vi "401_Audit_Report.vi"() -> (0 "error Out":errorcluster)   [LabVIEW 2015]
uses:
  Utilities/TypeDefs/401_Audit_Activity.ctl
  Utilities/TypeDefs/401_Audit_States.ctl
  <vilib>/addons/database/Connection.llb/Conn ObjectReference.ctl
  System Settings/Modules/LV2GActions.ctl
  <vilib>/Utility/miscctls.llb/LVPointTypeDef.ctl
  <vilib>/Utility/miscctls.llb/LVRowAndColumnUnsignedTypeDef.ctl
  <vilib>/addons/database/NI_Database_API.lvlib
panel:
  in  "Decending":bool caption="Asc/Des"
  in  "Tab Processing":enum32{"Page 1"}(tab)
  in  "VS":bool=TRUE
  in  "Export":bool
  in  "Tab Control":enum32{"Date", "User Name"}(tab)
  in  "Start Date":timestamp format="%<%H:%M:%S\n%Y/%m/%d>T"
  in  "End Date":timestamp format="%<%H:%M:%S\n%Y/%m/%d>T"
  in  "User":u16(ring) items=["Admin", "Supervisor", "Operator"]
  in  "Save":bool
  in  "Multicolumn Listbox":i32(listbox)
  in  "Activity":T1=enum."User show functionality for Info"
  in  "Previous Value":dbl
  in  "Current Value":dbl
  out "Date,Time":string
  in  "USER ID":string="Rahul"
  in  "Back":bool
  in  "Boolean":bool
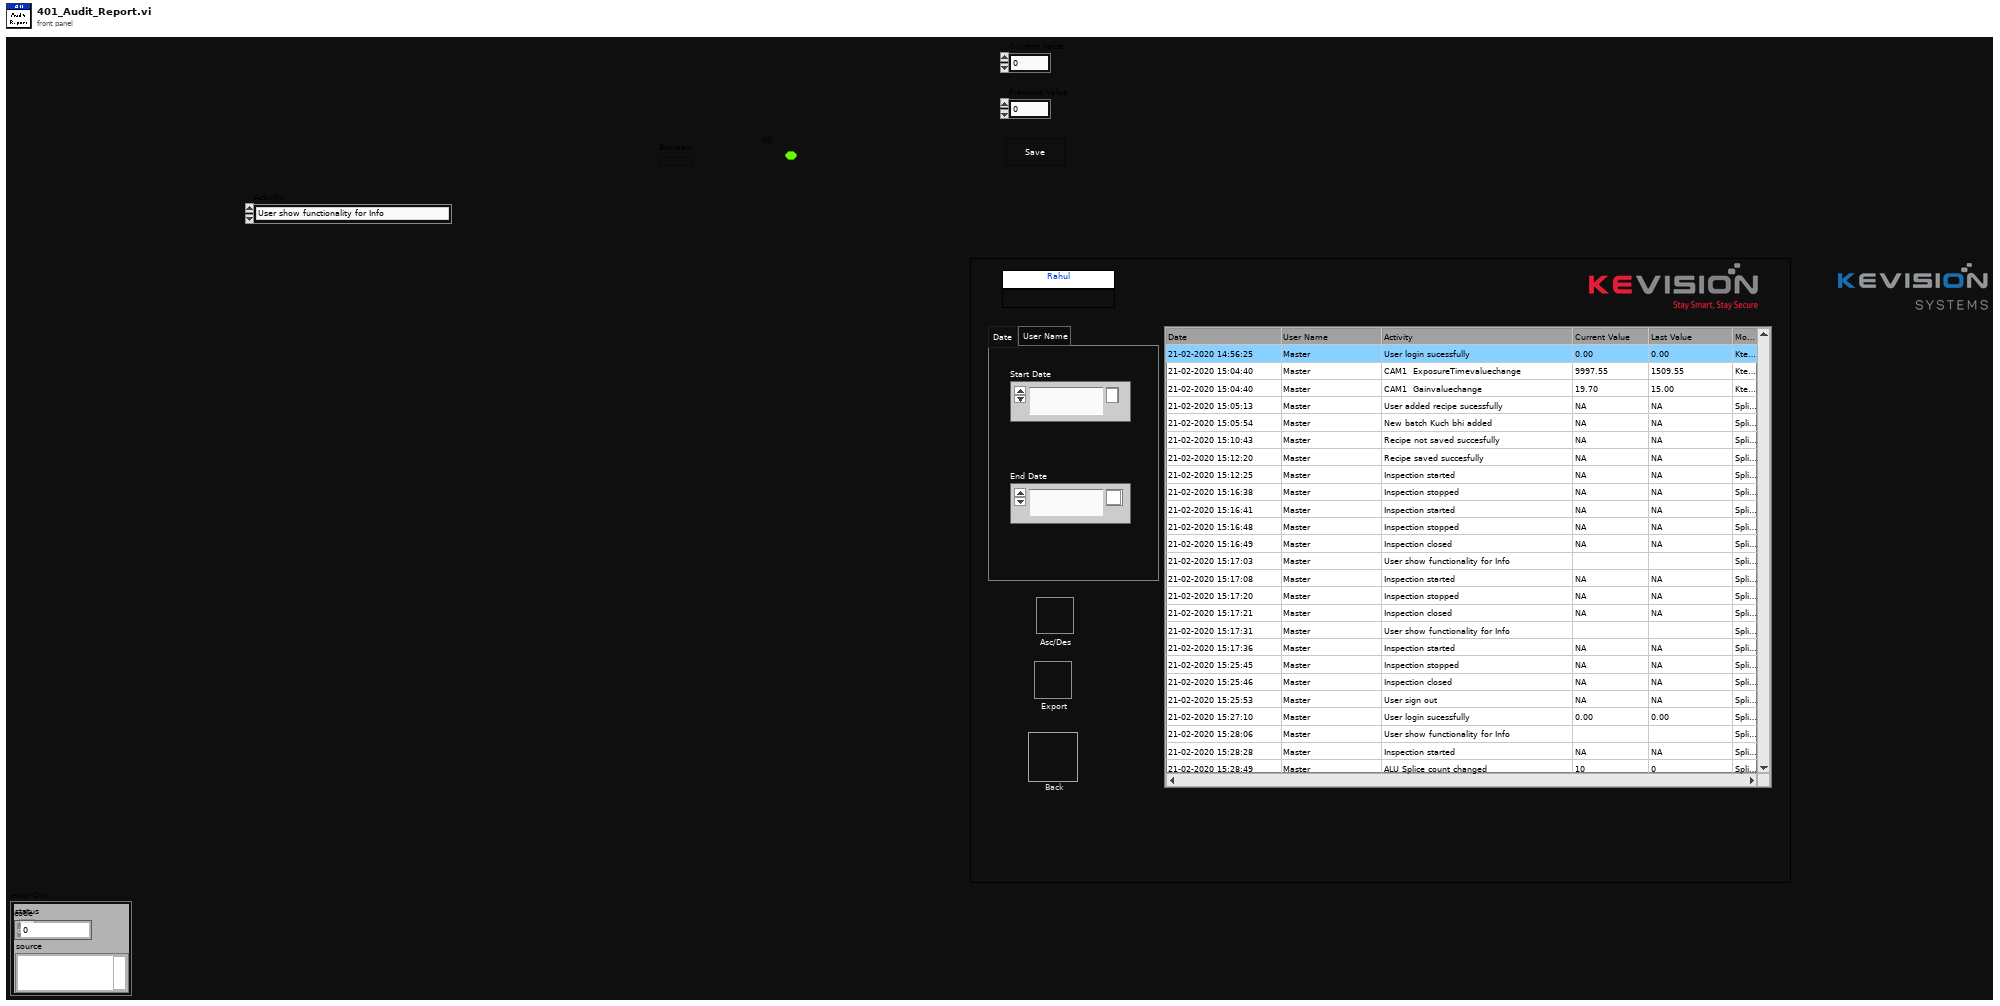
[diagram p1: front panel]
types:
  T1 = typedef "401_Audit_Activity.ctl" = enum16{"User login sucessfully", "User login fail", "User lock", "User sign out", "User added succesfully", "User edit succesFully", "User delete succesfully", "Reset password", "Forgot Password", "User change security policy", "User change user rights", "User allowed functionality for inspection", "User allowed  functionality for recipe", "User allowed functionality for teach", "User allowed  for user management", "User allowed for camera settings", "User allowed functionality for Hardware Check", "User allowed functionality for printer settings", "User allowed functionality for server settings", "User allowed  for third party settings", "User allowed  for System settings", "User allowed functionality For Test I/O", "User allowed and show functionality For Fault Images", "User allowed functionality for Production Report", "User allowed functionality for Audit Report", "User allowed functionality for Help", "User allowed functionality for  Info", "User show functionality for Inspection", "User show functionality for Teach", "User show functionality for Recipe", "User show functionality for User Management", "User show functionality for Camera Settings", "User show functionality for Hardware Check", "User show functionality for printer Settings", "User show functionality  for Server Settings", "User show functionality for Third party Settings", "User show functionality for System settings", "User show functionality for Test I/O", "User show functionality for Fault Images", "User show functionality for Production Report", "User show functionality for Audit Report", "User show functionality for Help", "User show functionality for Info", "User update Security Policy", "User added Recipe sucessfully", "User delete Recipe sucessfully", "User rename Recipe sucessfully", "User save Camera Settings sucessfully ", "User Close with out save", "User change Brightness", "User change Exposure Time", "User change Gain Value", "User change Saturation", "User change Gamma", "User change Sharpness", "User change Hue", "User change White Balance", "User change  Comport ", "User save Test I/o settings sucessfully", "User close with out saving ", "User change Light Timing ", "User change Light Flash ", "Camera Ready", "User change Inactive Period ", "User change Grab Delay", "User change Timed Output", "User change No Of Track", "User change Output Polarity ", "User chnage Output Timing", "User change Track Output ", "User Taught sucessfully", "User close with out  Taught.", "User could not able To Add User", "User could not Delete", "User could not Updated", "User could not change Security Policy", "User could not change User Rights"}
  T2 = typedef "401_Audit_States.ctl" = enum16{"Intialize", "UpdateControls", "Save", "User Interface", "Finalize", "View User Data", "View Date time Data", "Add Audit Data", "Decending", "Ascending", "Export To Html", "UpdateFPCControls", "Quit"}
  T3 = typedef "NI_Database_API.lvlib/Conn ObjectReference.ctl" = refnum<k1>
  T4 = cluster{"states":T2, "error in":cluster{"status":bool, "Error in":i32, "source":string}, "Save Data":cluster{"Current Value":dbl, "Previous Value":dbl, "Activity Name":string, "Camera Name":string}, "DB_Ref_In":T3, "Multicolumn Listbox":refnum<vi>, "Read Data":string[][], "Selecteduser":string}
  T5 = typedef "LV2GActions.ctl" = enum16{"Read", "Write", "Current", "Update", "UpdateSystemSettings", "UpdateModel"}
  T6 = typedef "LVPointTypeDef.ctl" = cluster{"Horizontal":i16, "Vertical":i16}
  T7 = cluster{"UserName":string, "Group Level":u16, "Theme":u16, "Software Type":u16, "System Language":u16, "Master":bool, "Recipe":string, "Batch":string, "Simulate":bool, "Trigger Activation":u16, "DateFormat":u16, "HardwareTest":bool}
  T8 = enum8{"Enabled", "Disabled", "Disabled and Grayed Out"}
  T9 = typedef "LVRowAndColumnUnsignedTypeDef.ctl" = cluster{"Row":u32, "Column":u32}
  T10 = enum16{"Read", "Current", "UpdateRecipiePath", "UpdateBatchPath"}
  T11 = cluster{"status":bool, "Error in":i32, "source":string}
  T12 = cluster{"BasePath":path, "RecipiePath":path, "BatchPath":path}
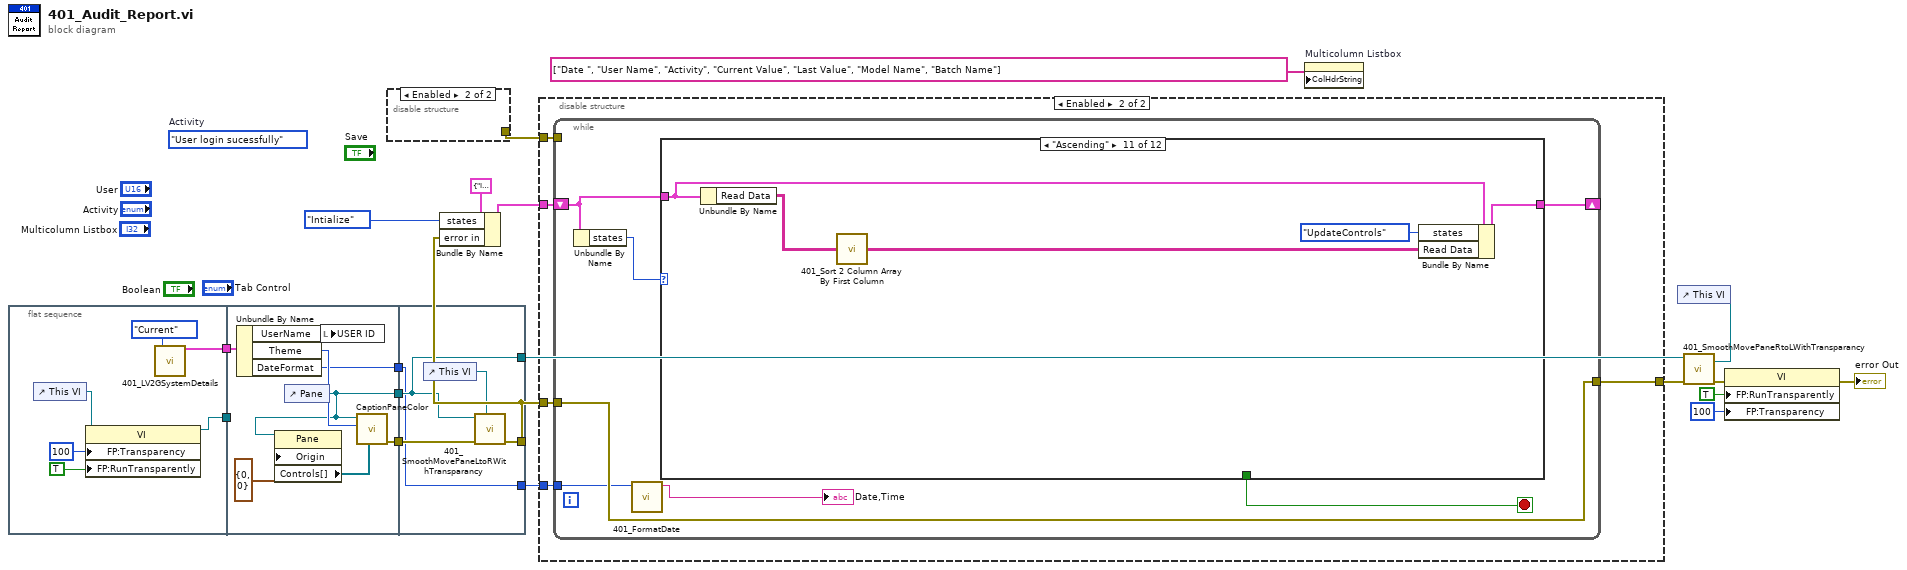
[diagram p0: block diagram]
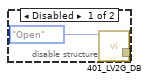
[diagram p2: hidden frame]
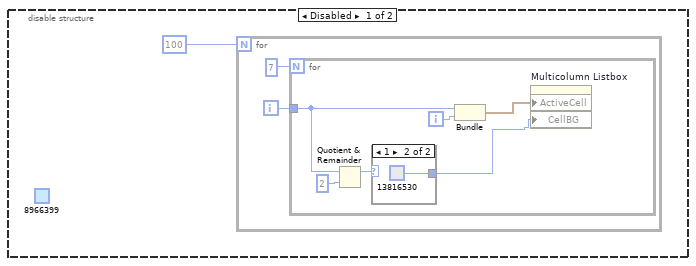
[diagram p3: hidden frame]
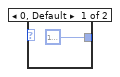
[diagram p4: hidden frame]
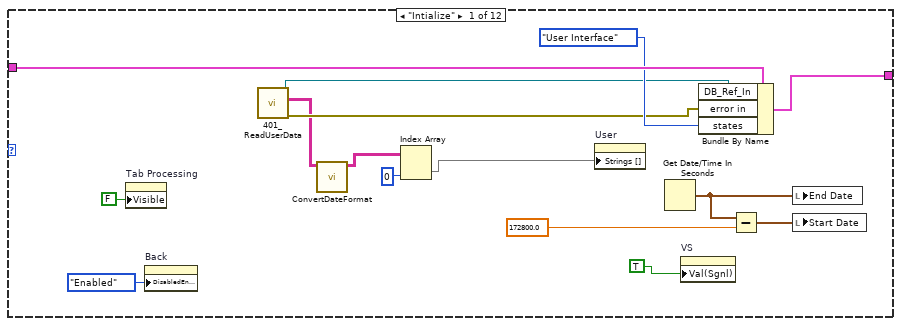
[diagram p5: hidden frame]
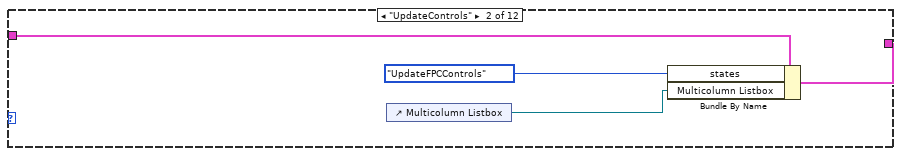
[diagram p6: hidden frame]
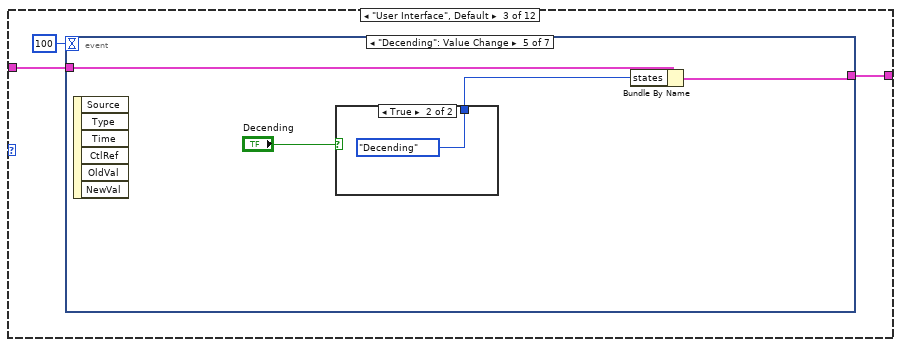
[diagram p7: hidden frame]
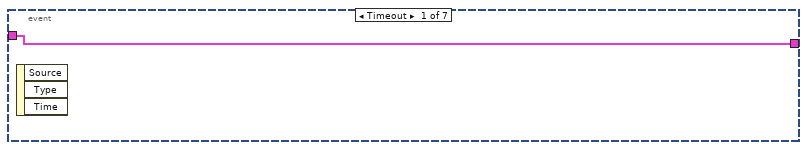
[diagram p8: hidden frame]
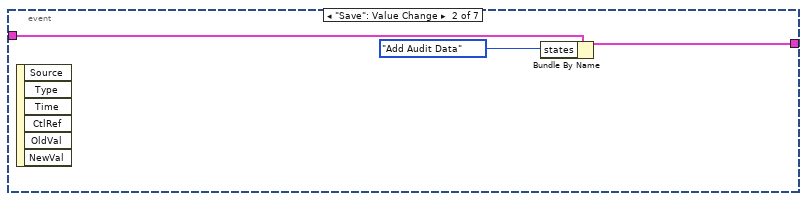
[diagram p9: hidden frame]
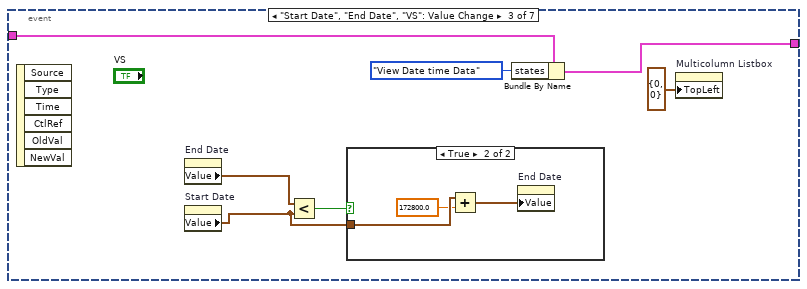
[diagram p10: hidden frame]
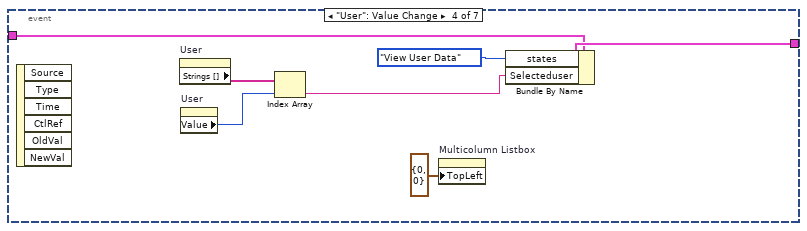
[diagram p12: hidden frame]
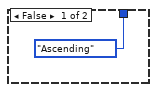
[diagram p13: hidden frame]
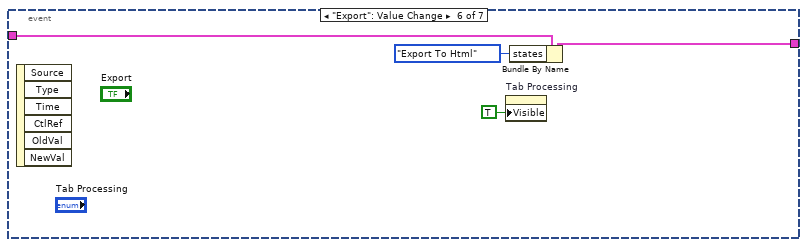
[diagram p14: hidden frame]
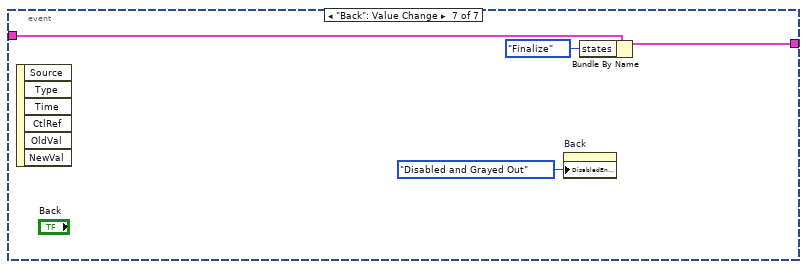
[diagram p15: hidden frame]
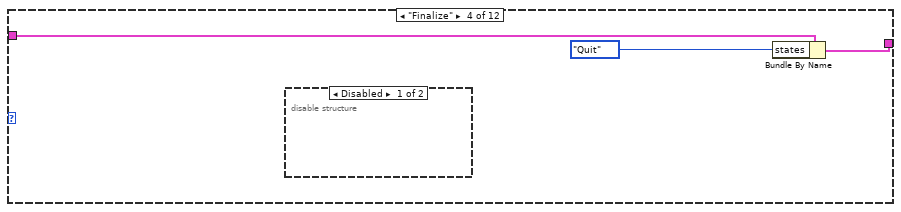
[diagram p16: hidden frame]
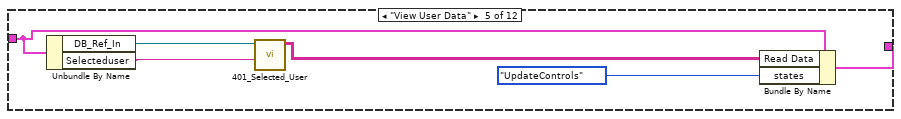
[diagram p18: hidden frame]
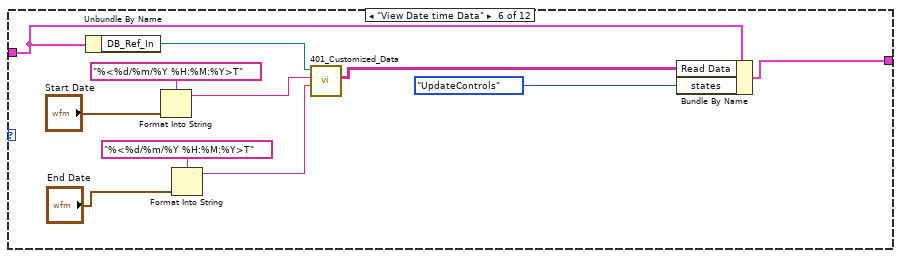
[diagram p19: hidden frame]
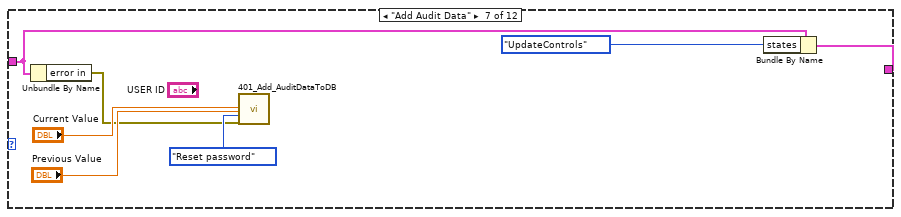
[diagram p20: hidden frame]
diagram:
  (unwired) 401_Audit_Activity."User login sucessfully"  # Activity
  n1 = flat-sequence {
    tunnel: [w22] -> w13
    tunnel: [w20] -> w11
    tunnel: w13 -> [_]
    tunnel: [w33] -> w12
    tunnel: w11 -> [w30]
    tunnel: [w27] -> w5
    tunnel: [w26] -> w2
    tunnel: [w37] -> w8
    tunnel: w12 -> [w36]
    tunnel: w5 -> [w35]
    tunnel: [w35] -> w4
    tunnel: [w34] -> w3
    tunnel: w2 -> [w34]
    frame #0 {
      n2 = control-ref of="This VI"() -> (w25:refnum<vi>)
      n3 = property class="VI"(reference=w25, "FP:Transparency"=u8 100 ("Front Panel Window:Transparency"), "FP:RunTransparently"=TRUE ("Front Panel Window:Run VI Transparently")) -> (reference out=w22:refnum<vi>)  [unwired: 1 in, 1 out]
      n4 = call "401_LV2GSystemDetails.vi"("R/W/C"=LV2GActions."Current") -> ("DataOut"=w20:T7)  [unwired: 17 in, 1 out]
    }
    frame #1 {
      n5 = Unbundle By Name(w30) -> ("UserName"=w28:string, "Theme"=w29:u16, "DateFormat"=w26:u16)
      n6 = control-ref of="Pane"() -> (w27:refnum<vi>)
      n7 = property class="Pane"(reference=w27, "Origin"=T6 {"Horizontal"=0, "Vertical"=0}) -> ("Controls[]"=w32:refnum<vi>[])  [unwired: 1 in, 2 out]
      n8 = local write "USER ID"(w28) -> ()
      n9 = call "CaptionPaneColor.vi"("Controls[]"=w32, "NewVal"=w29, "Pane in"=w27) -> ("error out"=w33:errorcluster)  [unwired: 8 in]
    }
    frame #2 {
      n10 = control-ref of="This VI"() -> (w38:refnum<vi>)
      n11 = call "401_SmoothMovePaneLtoRWithTransparancy.vi"("VI in"=w38, "error in (no error)"=w36, "Pane in"=w35) -> ("error out"=w37:errorcluster)  [unwired: 7 in, 1 out]
    }
  }
  n12 = disable-structure shown="Enabled" {
    disable-tunnel: [w39 _] -> w1
    frame Disabled {
      n13 = call "401_LV2G_DB.vi"("Action"=enum16{"Open", "Read", "Close"}."Open") -> ("error out"=w39:errorcluster)  [unwired: 9 in, 1 out]
    }
    frame Enabled {
    }
  }
  n14 = Bundle By Name(cluster=T4 {"states"=enum."Intialize", "error in"={"status"=FALSE, "Error in"=0, "source"=""}, "Save Data"={"Current Value"=0.0, "Previous Value"=0.0, "Activity Name"="", "Camera Name"=""}, "DB_Ref_In"=refnum, "Multicolumn Listbox"=refnum, "Read Data"=[], "Selecteduser"=""} ("input cluster"), "states"=401_Audit_States."Intialize", "error in"=w8) -> (w14:T4)
  n15 = disable-structure shown="Enabled" {
    disable-tunnel: w14 -> [_ w56]
    disable-tunnel: w8 -> [_ w55]
    disable-tunnel: [_ w54] -> w17
    disable-tunnel: w3 -> [_ w53]
    disable-tunnel: w1 -> [_ w52]
    frame Disabled {
      (unwired) u32 8966399
      n16 = for {
        N: 100 -> [_]
        i -> [w42]
        n17 = for {
          N: 7 -> [_]
          tunnel: w42 -> [w48]
          i -> [w49]
          n18 = Quotient & Remainder(x=w48, y=2) -> (x-y*floor(x/y)=w46:i32)  [unwired: 1 out]
          n19 = case shown="1" w46 {
            tunnel: [u32 16777226 u32 13816530] -> w45
            frame 0, Default {
            }
            frame 1 {
            }
          }
          n20 = Bundle(w48, w49) -> (w44:cluster{i32, i32})  [unwired: 1 in]
          n21 = property on="Multicolumn Listbox" class="MCListbox (strict)"("ActiveCell"=w44, "CellBG"=w45) -> ()  [unwired: 2 in, 2 out]
        }
      }
    }
    frame Enabled {
      n22 = while {
        shift-right: [w61] -> _
        shift-left: w56 -> [w60]
        tunnel: w55 -> [w63]
        tunnel: [w63] -> w54
        tunnel: w53 -> [w57]
        tunnel: w52 -> [_]
        stop <- w59 stop-if-true
        n23 = Unbundle By Name(w60) -> ("states"=w62:T2)
        n24 = call "401_FormatDate.vi"("DateFormat"=w57) -> ("date/time string"=→"Date,Time":string)  [unwired: 10 in]
        n25 = case shown="\"Ascending\"" w62 {
          tunnel: [w68 w81 w84 w123 w127 w139 w147 w152 w168 _ w177 w183] -> w61
          tunnel: w60 -> [w78 w82 w83 w121 w126 w140 w141 w150 w166 _ w176 w182]
          tunnel: [_ _ _ _ _ _ _ _ _ TRUE _ _] -> w59
          frame "Intialize" {
            n26 = property on="Tab Processing" class="TabCtl (strict)"("Visible"=FALSE) -> ()  [unwired: 2 in, 2 out]
            n27 = property on="Back" class="Bool"("DisabledEnum"=T8."Enabled" ("Disabled")) -> ()  [unwired: 2 in, 2 out]
            n28 = call "401_ReadUserData.vi"() -> ("error out"=w67:errorcluster, "User_Data"=w66:string[][], "Refnum out"=w69:T3)  [unwired: 9 in]
            n29 = call "ConvertDateFormat.vi"("DataIn"=w66) -> ("DataOut"=w65:string[][])  [unwired: 10 in]
            n30 = Index Array(array=w65, index (col)=0 ("disabled index (col)")) -> (element=w76:string[])  [unwired: 1 in]
            n31 = property on="User" class="Ring (strict)"("Strings []"=w76) -> ()  [unwired: 2 in, 2 out]
            n32 = Get Date/Time In Seconds() -> (seconds since 1Jan1904=w72:timestamp)
            n33 = property on="VS" class="Bool (strict)"("Val(Sgnl)"=TRUE ("Value (Signaling)")) -> ()  [unwired: 2 in, 2 out]
            n34 = Bundle By Name(cluster=w78, "DB_Ref_In"=w69, "error in"=w67, "states"=401_Audit_States."User Interface") -> (w68:T4)
            n35 = Subtract(x=w72, y=172800.0) -> (x-y=w73:timestamp)
            n36 = local write "End Date"(w72) -> ()
            n37 = local write "Start Date"(w73) -> ()
          }
          frame "UpdateControls" {
            n38 = control-ref of="Multicolumn Listbox"() -> (w79:refnum<vi>)
            n39 = Bundle By Name(cluster=w82, "states"=401_Audit_States."UpdateFPCControls", "Multicolumn Listbox"=w79) -> (w81:T4)
          }
          frame "User Interface", Default {
            n40 = event shown="[4] \"Decending\": Value Change" {
              selector: _ -> [_ _ _ _ _ _ _]
              dyn-events: _ -> [_ _ _ _ _ _ _]
              timeout: 100 -> [_ _ _ _ _ _ _]
              tunnel: [w86 w89 w96 w106 w110 w116 w120] -> w84
              tunnel: w83 -> [w86 w87 w95 w105 w109 w115 w119]
              event Timeout {
                n41 = event-data() -> ()  [unwired: 1 in, 3 out]
              }
              event "Save": Value Change {
                n42 = event-data() -> ()  [unwired: 1 in, 6 out]
                n43 = Bundle By Name(cluster=w87, "states"=401_Audit_States."Add Audit Data") -> (w89:T4)
              }
              event "Start Date", "End Date", "VS": Value Change {
                n44 = event-data() -> ()  [unwired: 1 in, 6 out]
                n45 = property on="End Date" class="AbsTime (strict)"() -> ("Value"=w92:timestamp)  [unwired: 2 in, 2 out]
                n46 = property on="Start Date" class="AbsTime (strict)"() -> ("Value"=w90:timestamp)  [unwired: 2 in, 2 out]
                n47 = Less?(x=w92, y=w90) -> (x < y?=w91:bool)
                n48 = case shown="True" w91 {
                  tunnel: w90 -> [_ w99]
                  frame False {
                  }
                  frame True {
                    n49 = Add(x=w99, y=172800.0) -> (x+y=w97:timestamp)
                    n50 = property on="End Date" class="AbsTime (strict)"("Value"=w97) -> ()  [unwired: 2 in, 2 out]
                  }
                }
                n51 = Bundle By Name(cluster=w95, "states"=401_Audit_States."View Date time Data") -> (w96:T4)
                n52 = property on="Multicolumn Listbox" class="MCListbox (strict)"("TopLeft"=T9 {"Row"=0, "Column"=0} ("Top Left Visible Cell")) -> ()  [unwired: 2 in, 2 out]
              }
              event "User": Value Change {
                n53 = event-data() -> ()  [unwired: 1 in, 6 out]
                n54 = property on="User" class="Ring (strict)"() -> ("Strings []"=w103:string[])  [unwired: 2 in, 2 out]
                n55 = property on="User" class="Ring (strict)"() -> ("Value"=w102:u16)  [unwired: 2 in, 2 out]
                n56 = Index Array(array=w103, index=w102) -> (element=w101:string)
                n57 = property on="Multicolumn Listbox" class="MCListbox (strict)"("TopLeft"=T9 {"Row"=0, "Column"=0} ("Top Left Visible Cell")) -> ()  [unwired: 2 in, 2 out]
                n58 = Bundle By Name(cluster=w105, "states"=401_Audit_States."View User Data", "Selecteduser"=w101) -> (w106:T4)
              }
              event "Decending": Value Change {
                n59 = event-data() -> ()  [unwired: 1 in, 6 out]
                n60 = case shown="True" "Decending" {
                  tunnel: [401_Audit_States."Ascending" ("states") 401_Audit_States."Decending" ("states")] -> w107
                  frame False {
                  }
                  frame True {
                  }
                }
                n61 = Bundle By Name(cluster=w109, "states"=w107) -> (w110:T4)
              }
              event "Export": Value Change {
                n62 = event-data() -> ()  [unwired: 1 in, 6 out]
                n63 = property on="Tab Processing" class="TabCtl (strict)"("Visible"=TRUE) -> ()  [unwired: 2 in, 2 out]
                n64 = Bundle By Name(cluster=w115, "states"=401_Audit_States."Export To Html") -> (w116:T4)
              }
              event "Back": Value Change {
                n65 = event-data() -> ()  [unwired: 1 in, 6 out]
                n66 = property on="Back" class="Bool"("DisabledEnum"=T8."Disabled and Grayed Out" ("Disabled")) -> ()  [unwired: 2 in, 2 out]
                n67 = Bundle By Name(cluster=w119, "states"=401_Audit_States."Finalize") -> (w120:T4)
              }
            }
          }
          frame "Finalize" {
            n68 = disable-structure shown="Disabled" {
              frame Disabled {
              }
              frame Enabled {
              }
            }
            n69 = Bundle By Name(cluster=w121, "states"=401_Audit_States."Quit") -> (w123:T4)
          }
          frame "View User Data" {
            n70 = Unbundle By Name(w126) -> ("DB_Ref_In"=w129:T3, "Selecteduser"=w128:string)
            n71 = call "401_Selected_User.vi"("User Name"=w128, "connection in"=w129) -> ("Data_Table"=w125:string[][])  [unwired: 8 in, 1 out]
            n72 = Bundle By Name(cluster=w126, "Read Data"=w125, "states"=401_Audit_States."UpdateControls") -> (w127:T4)
          }
          frame "View Date time Data" {
            n73 = Unbundle By Name(w140) -> ("DB_Ref_In"=w137:T3)
            n74 = Format Into String(format string="%<%d/%m/%Y %H:%M:%Y>T", "Start Date") -> (resulting string=w133:string)  [unwired: 2 in, 1 out]
            n75 = Format Into String(format string="%<%d/%m/%Y %H:%M:%Y>T", "End Date") -> (resulting string=w130:string)  [unwired: 2 in, 1 out]
            n76 = call "401_Customized_Data.vi"("End_date"=w130, "Start_date"=w133, "connection in"=w137) -> ("Data_Table"=w136:string[][])  [unwired: 6 in, 2 out]
            n77 = Bundle By Name(cluster=w140, "Read Data"=w136, "states"=401_Audit_States."UpdateControls") -> (w139:T4)
          }
          frame "Add Audit Data" {
            n78 = Unbundle By Name(w141) -> ("error in"=w142:T11)
            n79 = call "401_Add_AuditDataToDB.vi"("Current Value"="Current Value", "Previous Value"="Previous Value", "Activity"=401_Audit_Activity."Reset password", "error in (no error)"=w142) -> ()  [unwired: 23 in, 1 out]
            n80 = Bundle By Name(cluster=w141, "states"=401_Audit_States."UpdateControls") -> (w147:T4)
          }
          frame "UpdateFPCControls" {
            n81 = call "401_Update_audit_control.vi"("input cluster 2"=w150) -> ("error Out"=w148:errorcluster)  [unwired: 10 in]
            n82 = property on="Multicolumn Listbox" class="MCListbox (strict)"(error in=w148) -> ("ItemNames"=w157:string[][])  [unwired: 1 in, 2 out]
            n83 = call "401_LV2GFilePath.vi"("Read"=T10."Current") -> ("Path"=w153:T12)  [unwired: 17 in, 1 out]
            n84 = Unbundle By Name(w153) -> ("BasePath"=w158:path)
            n85 = Index Array(array=w157, index (col)=0 ("index (row)")) -> (element=w156:string[])  [unwired: 1 in]
            n86 = Strip Path(path=w158) -> (name=w155:string)  [unwired: 1 out]
            n87 = Search 1D Array(1D array=w156, element=w155) -> (index of element=w149:i32)  [unwired: 1 in]
            n88 = property on="Multicolumn Listbox" class="MCListbox (strict)"("Val(Sgnl)"=w149, "Value"=w149) -> ()  [unwired: 2 in, 2 out]
            n89 = Bundle By Name(cluster=w150, "states"=401_Audit_States."User Interface") -> (w152:T4)
          }
          frame "Export To Html" {
            n90 = Unbundle By Name(w166) -> ("Read Data"=w160:string[][])
            n91 = property on="Multicolumn Listbox" class="MCListbox (strict)"() -> ("ColHdrString"=w165:string[])  [unwired: 2 in, 2 out]
            n92 = call "401_Read_Formate.vi"("Action"=enum16{"Read", "Write"}."Read") -> ("Numeric"=w163:i32)  [unwired: 9 in, 1 out]
            n93 = case shown="1" w163 {
              tunnel: [enum16{"HTML", "PDF"}."HTML" ("Enum") enum16{"HTML", "PDF"}."PDF" ("Enum")] -> w161
              frame 0, Default {
              }
              frame 1 {
              }
            }
            n94 = call "401_Export_ Report_Html.vi"("Enum"=w161, "Data"=w160, "column headers"=w165) -> ("Error out"=w164:errorcluster)  [unwired: 16 in]
            n95 = flat-sequence {
              tunnel: w164 -> [_]
              frame #0 {
                n96 = Wait (ms)(milliseconds to wait=u32 2000) -> ()  [unwired: 1 out]
              }
              frame #1 {
                n97 = property on="Tab Processing" class="TabCtl (strict)"("Visible"=FALSE) -> ()  [unwired: 2 in, 2 out]
              }
            }
            n98 = Bundle By Name(cluster=w166, "states"=401_Audit_States."User Interface") -> (w168:T4)
          }
          frame "Quit" {
          }
          frame "Ascending" {
            n99 = Unbundle By Name(w176) -> ("Read Data"=w178:string[][])
            n100 = call "401_Sort 2 Column Array By First Column.vi"("Data_Table"=w178) -> ("Array"=w175:string[][])
            n101 = Bundle By Name(cluster=w176, "states"=401_Audit_States."UpdateControls", "Read Data"=w175) -> (w177:T4)
          }
          frame "Decending" {
            n102 = Unbundle By Name(w182) -> ("Read Data"=w180:string[][])
            n103 = call "401_decending.vi"("Data_Table"=w180) -> ("Array"=w179:string[][])  [unwired: 10 in]
            n104 = Bundle By Name(cluster=w182, "states"=401_Audit_States."UpdateControls", "Read Data"=w179) -> (w183:T4)
          }
        }
      }
    }
  }
  n105 = property on="Multicolumn Listbox" class="MCListbox (strict)"("ColHdrString"=string[] ["Date ", "User Name", "Activity", "Current Value", "Last Value", "Model Name", "Batch Name"] ("Column Header Strings[]")) -> ()  [unwired: 2 in, 2 out]
  n106 = control-ref of="This VI"() -> (w6:refnum<vi>)
  n107 = call "401_SmoothMovePaneRtoLWithTransparancy.vi"("This VI"=w6, "error in"=w17, "Pane in"=w4) -> ("error out"=w16:errorcluster)  [unwired: 7 in, 1 out]
  n108 = property class="VI"(error in=w16, "FP:RunTransparently"=TRUE ("Front Panel Window:Run VI Transparently"), "FP:Transparency"=u8 100 ("Front Panel Window:Transparency")) -> (error out=→"error Out":errorcluster)  [unwired: 1 in, 1 out]
